vi "AdjustPower.vi"(0 "object in":refnum<class "InstrumentBase.lvclass">, 2 "DesiredPower(W)":dbl, 5 "error in (no error)":errorcluster) -> (14 "object out":refnum<class "InstrumentBase.lvclass">, 19 "error out":errorcluster)   [LabVIEW 2019, in "InstrumentBase.lvclass"]
uses:
  InstrumentBase.lvclass
  InstrumentBase.lvclass/InstrumentBase.ctl
panel:
  out "AmplitudeOk":bool
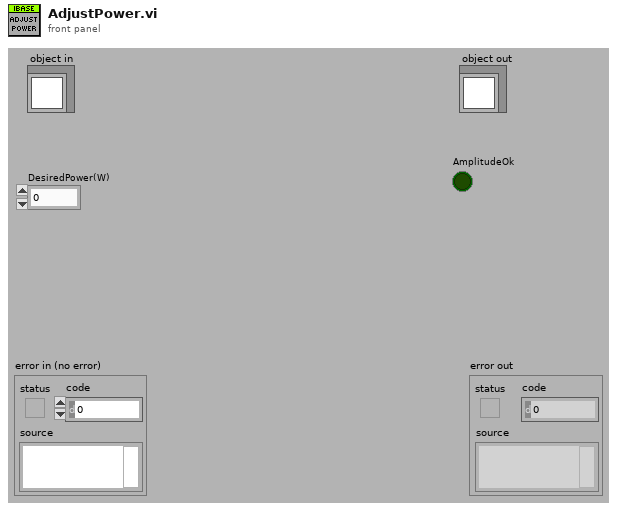
[diagram p1: front panel]
types:
  T1 = cluster{"Ch1.Carrier.Amplitude (V)":dbl, "Ch2.Carrier.Amplitude(V)":dbl}
  T2 = cluster{"Config.Ch1.Carrier.Frequency (Hz)":dbl, "Config.Ch2.Carrier.Frequency (Hz)":dbl, "Config.Ch1.Carrier.Amplitude (V)":dbl, "Config.Ch2.Carrier.Amplitude (V)":dbl}
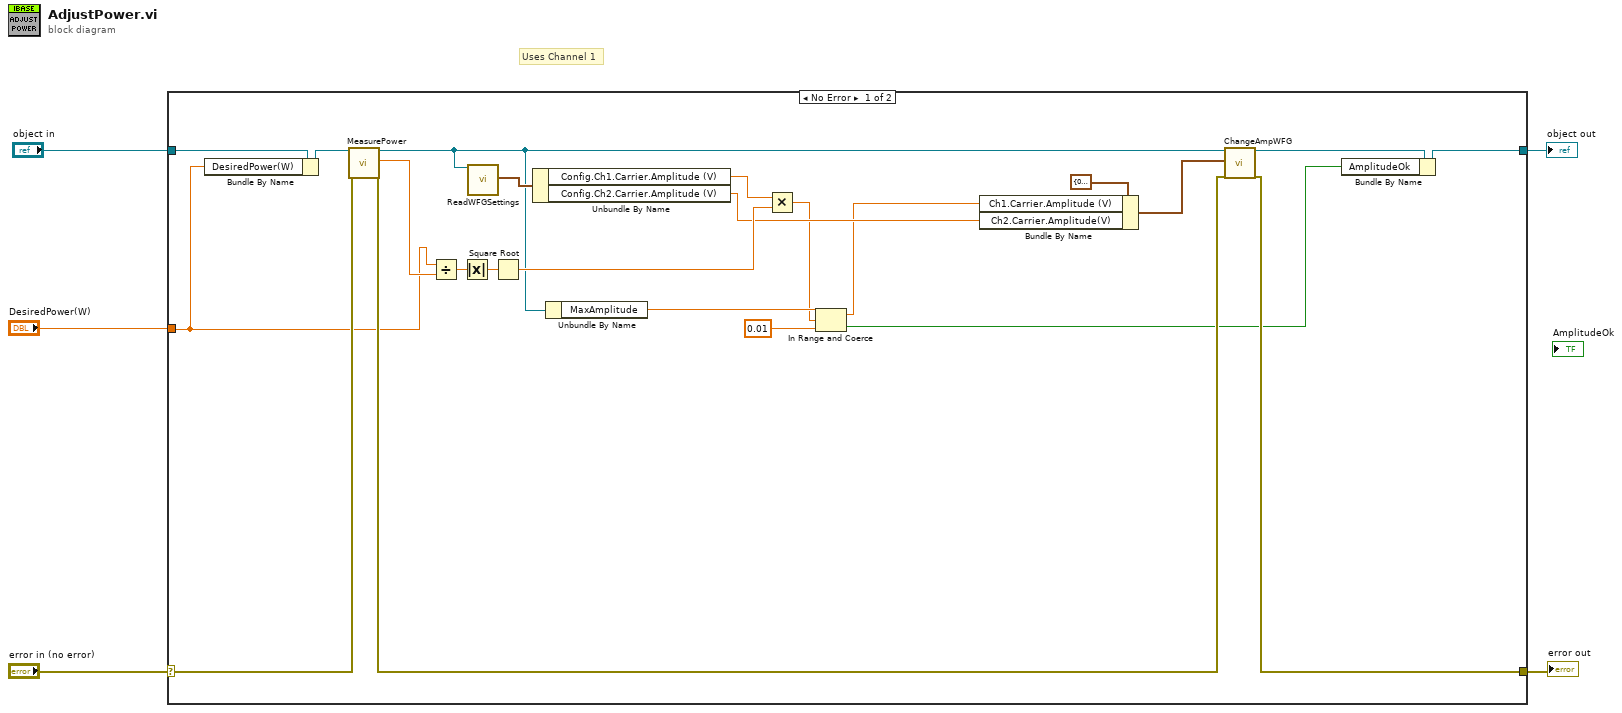
[diagram p0: block diagram]
diagram:
  # "Uses Channel 1"
  n1 = case shown="No Error" "error in (no error)" {
    selector: "error in (no error)" -> [w27 w30]
    tunnel: [w16 w30] -> w4
    tunnel: [w12 w29] -> w2
    tunnel: "object in" -> [w28 w29]
    tunnel: "DesiredPower(W)" -> [w6 _]
    frame No Error {
      n2 = Bundle By Name(cluster=w28, "DesiredPower(W)"=w6) -> (w7:refnum<class "InstrumentBase.lvclass">)
      n3 = call-dynamic "MeasurePower.vi"("object in"=w7, "error in (no error)"=w27) -> ("object out"=w15:refnum<class "InstrumentBase.lvclass">, "Measured Power"=w25:dbl, "error out"=w17:errorcluster)  [unwired: 14 in, 1 out]
      n4 = Divide(x=w6, y=w25) -> (x/y=w24:dbl)
      n5 = Absolute Value(x=w24) -> (abs(x)=w8:dbl)
      n6 = call-dynamic "ReadWFGSettings.vi"("object in"=w15) -> ("AmplitudeAndVoltage"=w21:T2)  [unwired: 16 in, 2 out]
      n7 = Square Root(x=w8) -> (sqrt(x)=w23:dbl)
      n8 = Unbundle By Name(w21) -> ("Config.Ch1.Carrier.Amplitude (V)"=w22:dbl, "Config.Ch2.Carrier.Amplitude (V)"=w20:dbl)
      n9 = Unbundle By Name(w15) -> ("MaxAmplitude"=w14:dbl)
      n10 = Multiply(x=w22, y=w23) -> (x*y=w10:dbl)
      n11 = In Range and Coerce(upper limit=w14, x=w10, lower limit=0.01) -> (coerced(x)=w9:dbl, In Range?=w11:bool)
      n12 = Bundle By Name(cluster=T1 {"Ch1.Carrier.Amplitude (V)"=0.0, "Ch2.Carrier.Amplitude(V)"=0.0} ("AmplitudeCh1&2"), "Ch1.Carrier.Amplitude (V)"=w9, "Ch2.Carrier.Amplitude(V)"=w20) -> (w19:T1)
      n13 = call-dynamic "ChangeAmpWFG.vi"("object in"=w15, "AmplitudeCh1&2"=w19, "error in (no error)"=w17) -> ("object out"=w18:refnum<class "InstrumentBase.lvclass">, "error out"=w16:errorcluster)  [unwired: 15 in]
      n14 = Bundle By Name(cluster=w18, "AmplitudeOk"=w11) -> (w12:refnum<class "InstrumentBase.lvclass">)
    }
    frame Error {
    }
  }
  "error out" <- w4
  "object out" <- w2
